vi "Stop Work.vi"(8 "error in (no error)":errorcluster, 9 "Reply":bool=TRUE, 10 "Reply to":refnum<class "Stop Response Msg.lvclass">, 11 "Measure Object in":refnum<class "Worker.lvclass">) -> (0 "error out":errorcluster, 3 "Measure Object out":refnum<class "Worker.lvclass">)   [LabVIEW 2016, in "Worker.lvclass"]
uses:
  Worker/Worker.lvclass
  C:/github/LabActor/Template Module/Template Module.lvclass
  Controllers/Process Controller Messages/Stop Response Msg/Stop Response Msg.lvclass
  Worker/Worker State.ctl
  Worker/Worker.lvclass/Worker.ctl
  Template Module.lvclass/Template Module.ctl
  Controllers/Process Controller Messages/Stop Response Msg/Stop Response Msg.lvclass/Stop Response Msg.ctl
  Controllers/Process Controller Messages/Stop Response Msg/Write Name.vi
  Write State.vi
  Read Name.vi
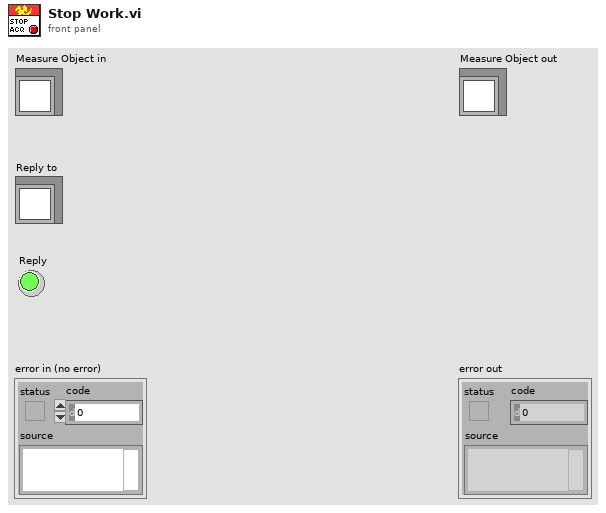
[diagram p1: front panel]
types:
  T1 = typedef "Worker State.ctl" = enum16{"Idle", "Starting", "Working", "Stopping"}
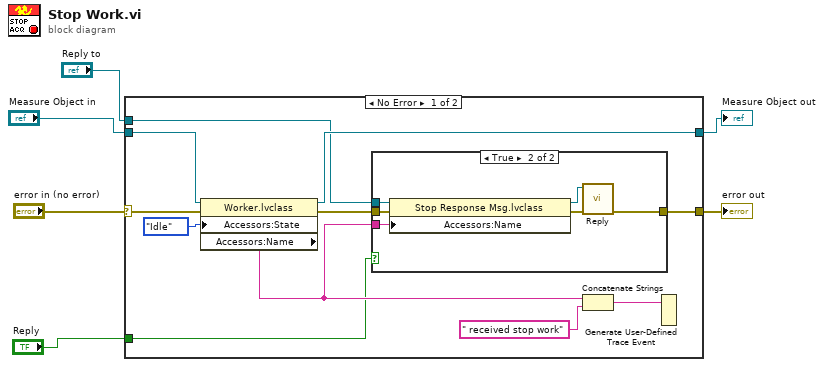
[diagram p0: block diagram]
diagram:
  n1 = case shown="No Error" "error in (no error)" {
    selector: "error in (no error)" -> [w15 w26]
    tunnel: [w8 w26] -> w5
    tunnel: [w16 w25] -> w3
    tunnel: "Measure Object in" -> [w17 w25]
    tunnel: "Reply to" -> [w11 _]
    tunnel: "Reply" -> [w7 _]
    frame No Error {
      n2 = property class="Worker.lvclass"(reference=w17, error in=w15, "Accessors:State"=Worker_State."Idle" ("State")) -> (reference out=w16:refnum<class "Worker.lvclass">, error out=w9:errorcluster, "Accessors:Name"=w10:string)
      n3 = case shown="True" w7 {
        tunnel: w11 -> [_ w24]
        tunnel: w10 -> [_ w23]
        tunnel: w9 -> [w18 w22]
        tunnel: [w18 w19] -> w8
        frame False {
        }
        frame True {
          n4 = property class="Stop Response Msg.lvclass"(reference=w24, error in=w22, "Accessors:Name"=w23) -> (reference out=w21:refnum<class "Stop Response Msg.lvclass">, error out=w20:errorcluster)
          n5 = call-dynamic "Reply.vi"("error in (no error)"=w20, "Self-addressed Msg in"=w21) -> ("error out"=w19:errorcluster)  [unwired: 8 in, 1 out]
        }
      }
      n6 = Concatenate Strings(w10, " received stop work" ("string")) -> (w13:string)
      n7 = Generate User-Defined Trace Event(2:w13) -> ()  [unwired: 1 in]
    }
    frame Error {
    }
  }
  "error out" <- w5
  "Measure Object out" <- w3
